vi "array exercise.vi"() -> ()   [LabVIEW 2016]
panel:
  out "Mid Array Value":dbl
  out "Final Array":dbl[](array[numeric])
  in  "Terminal Array":dbl[](array[numeric])
  in  "Element 2":dbl
  in  "Element 1":dbl
  in  "Initial Array":dbl[](array[numeric])
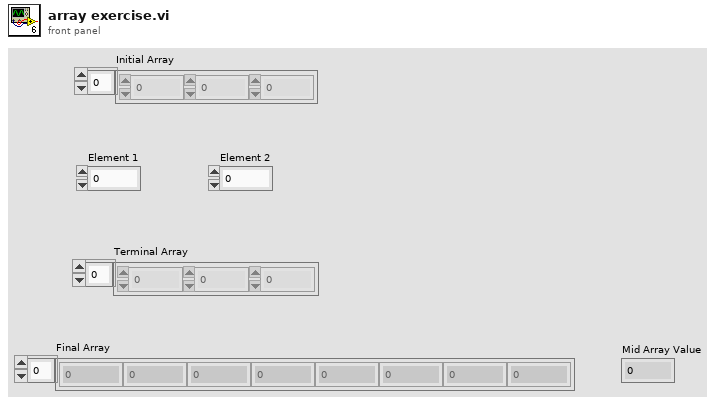
[diagram p1: front panel]
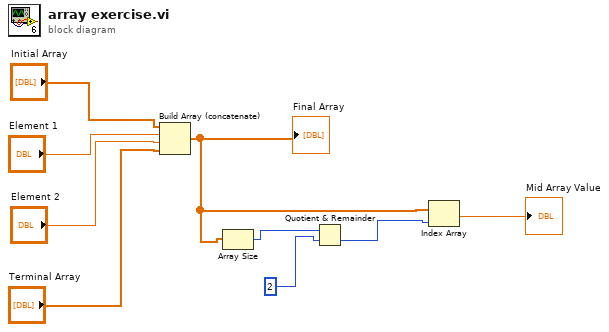
[diagram p0: block diagram]
diagram:
  n1 = Build Array (concatenate)("Initial Array", "Element 1", "Element 2", "Terminal Array") -> (w5:dbl[])
  "Final Array" <- w5
  n2 = Array Size(array=w5) -> (size(s)=w3:i32)
  n3 = Quotient & Remainder(x=w3, y=2) -> (floor(x/y)=w1:i32)  [unwired: 1 out]
  n4 = Index Array "Index Array"(array=w5, index=w1) -> (element=→"Mid Array Value":dbl)
